vi "WinClipCursor.vi"(8 "error in (no error)":errorcluster, 11 "RECT":T1) -> (0 "error out":errorcluster)   [LabVIEW 2021, in "RocketPlot.lvlib"]
uses:
  RocketPlot.lvlib
  USER32.DLL
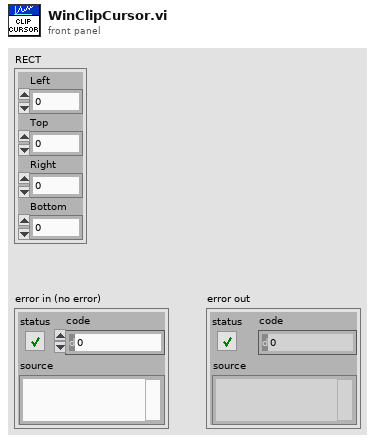
[diagram p1: front panel]
types:
  T1 = cluster{"Left":i32, "Top":i32, "Right":i32, "Bottom":i32}
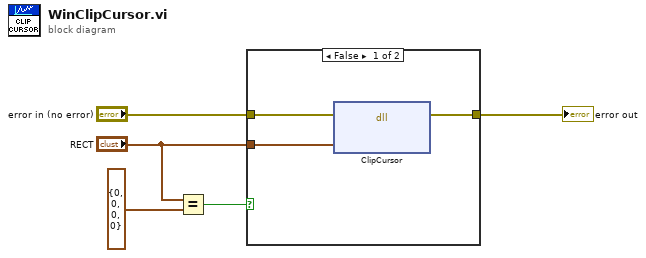
[diagram p0: block diagram]
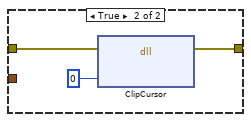
[diagram p2: hidden frame]
diagram:
  n1 = Equal?(x="RECT", y=T1 {"Left"=0, "Top"=0, "Right"=0, "Bottom"=0} ("RECT")) -> (x = y?=w1:bool)
  n2 = case shown="False" w1 {
    tunnel: "RECT" -> [w8 _]
    tunnel: "error in (no error)" -> [w7 w11]
    tunnel: [w6 w10] -> w2
    frame False {
      n3 = dll-call lib="user32.dll" fn="ClipCursor"(error in=w7, "RECT"=w8) -> (error out=w6:errorcluster)  [unwired: 3 in, 2 out]
    }
    frame True {
      n4 = dll-call lib="user32.dll" fn="ClipCursor"(error in=w11, "RECT"=0) -> (error out=w10:errorcluster)  [unwired: 3 in, 2 out]
    }
  }
  "error out" <- w2
